vi "Beta PDF.vi"(9 "b":dbl=4.0, 10 "a":dbl=2.0, 11 "x":dbl=0.5) -> (0 "error":i32, 3 "pdf(x)":dbl=1.2499999999999998)   [LabVIEW 2020, in "NI_Gmath.lvlib"]
doc: "Computes the continuous probability density function (PDF) of various distributions. You must manually select the polymorphic instance to use."
uses:
  NI_Gmath.lvlib
  st_error_code.ctl
panel:
  # "Beta PDF"
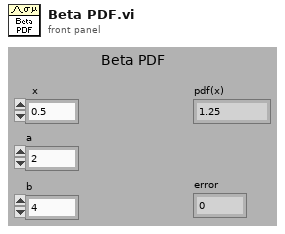
[diagram p1: front panel]
types:
  T1 = typedef "NI_Gmath.lvlib/st_error_code.ctl" = i32
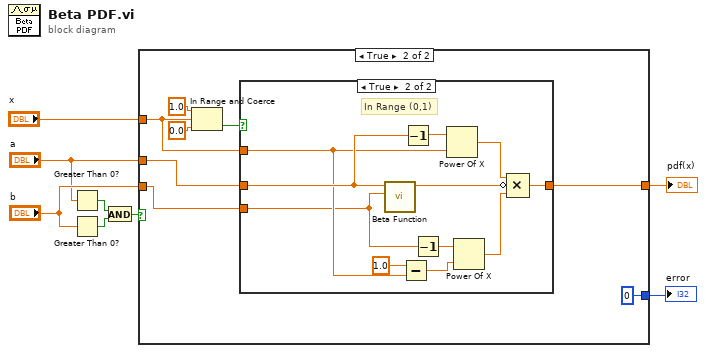
[diagram p0: block diagram]
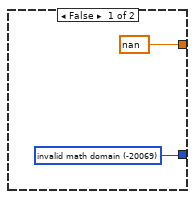
[diagram p2: hidden frame]
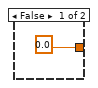
[diagram p3: hidden frame]
diagram:
  n1 = Greater Than 0?(x="a") -> (x > 0?=w1:bool)
  n2 = Greater Than 0?(x="b") -> (x > 0?=w2:bool)
  n3 = And(x=w1, y=w2) -> (x .and. y?=w3:bool)
  n4 = case shown="True" w3 {
    tunnel: "b" -> [_ w13]
    tunnel: [w9 0 ("invalid math domain")] -> w8
    tunnel: [nan w16] -> w7
    tunnel: "x" -> [_ w15]
    tunnel: "a" -> [_ w14]
    frame False {
      w9 = T1 -20069 items=["invalid math domain"=-20069, "Fourier interpolation size m >= n"=-20070, "empty array"=-20003] ("stat interp error code")
    }
    frame True {
      n5 = In Range and Coerce(upper limit=1.0, x=w15, lower limit=0.0) -> (In Range?=w17:bool)  [unwired: 1 out]
      n6 = case shown="True" w17 {
        tunnel: [0.0 w22] -> w16
        tunnel: w15 -> [_ w27]
        tunnel: w14 -> [_ w30]
        tunnel: w13 -> [_ w24]
        frame False {
        }
        frame True {
          # "In Range (0,1)"
          n7 = call "Beta Function.vi"("y"=w24, "x"=w30) -> ("b(x, y)"=w23:dbl)  [unwired: 9 in]
          n8 = Subtract(x=1.0, y=w27) -> (x-y=w25:dbl)
          n9 = Decrement(x=w30) -> (x-1=w29:dbl)
          n10 = Decrement(x=w24) -> (x-1=w26:dbl)
          n11 = Power Of X(1:w27, 2:w29) -> (0:w20:dbl)
          n12 = Power Of X(1:w25, 2:w26) -> (0:w21:dbl)
          n13 = Compound Arithmetic op=MULTIPLY(w20, invert w23, w21) -> (w22:dbl)
        }
      }
    }
  }
  "pdf(x)" <- w7
  "error" <- w8
